vi "AdjustCorrectPosition.vi"(6 "Robot":refnum<class "Robot.lvclass">, 7 "Game":refnum<class "Game.lvclass">, 8 "error in (no error)":errorcluster, 9 "IsShoot?":bool, 10 "Position":dbl[](array[numeric]), 11 "Utilities in":refnum<class "Utilities.lvclass">) -> (0 "error out":errorcluster, 1 "AdjustPosition":dbl[](array[numeric]), 3 "Utilities out":refnum<class "Utilities.lvclass">)   [LabVIEW 2021, in "Utilities.lvclass"]
uses:
  Utilities.lvclass
  Game_class/Game.lvclass
  Robot_class/Robot.lvclass
  Team_class/OffensivePlay.ctl
  Game_class/Game.lvclass/Game.ctl
  Parameters_class/Parameters.lvclass/Parameters.ctl
  Team_class/Team.lvclass/Team.ctl
  Object_class/Object.lvclass/Object.ctl
  Object_class/Read x.vi
  Object_class/Read y.vi
  Game_class/Read FieldRef.vi
  Game_class/Read EnemyRef.vi
  Game_class/Read BallRef.vi
  Game_class/Read Parameters.lvclass.vi
  Game_class/Read NewParameters.vi
  Game_class/Read OffensiveTeam.vi
  Team_class/Read OffensivePlay.vi
  Parameters_class/Read DistanceArea.vi
  Parameters_class/Read DistanceStop.vi
  Ally_class/Ally.lvclass
  Field_class/Field.lvclass
  Enemy_class/Enemy.lvclass
  Ball_class/Ball.lvclass
  Parameters_class/Parameters.lvclass
panel:
  out "output variable":sgl
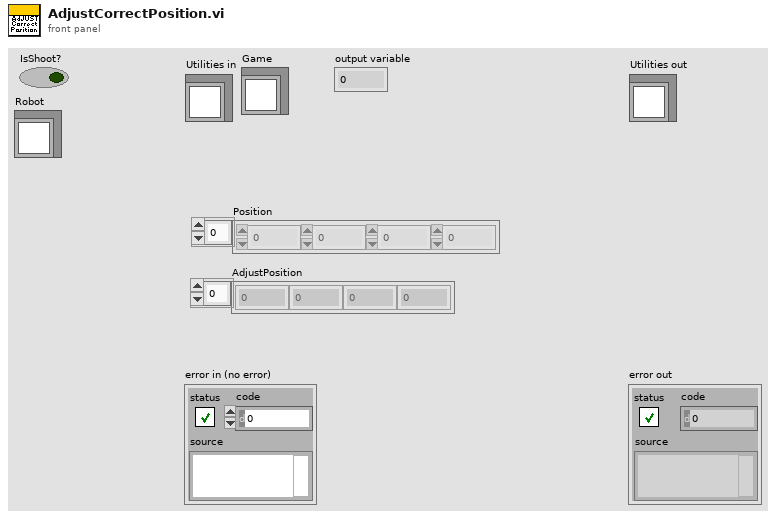
[diagram p1: front panel]
types:
  T1 = typedef "OffensivePlay.ctl" = enum16{"5RobotsPassGamePlay", "5PreparePassGame", "5RobotsKeeperGame", "KeeperPassToStriker", "5RobotsNormalGamePlay", "PrepareKeeperPass", "ACBPass", "ABCPass", "PrepareTriplePass", "TableWithStriker", "TableWith2ndStrikerPlay", "PrepareDoublePass", "PrepareRollToPass", "SimplePass", "PreparePass", "PassToStriker", "BallOutOfField", "PassTo2ndStriker", "StopOffensive", "Prepare Penalty Enemy", "EnemyPossessionAtEnemyField", "EnemyPossesionAtOurField", "TestPlay", "PreparePenaltyAlly", "KickPenaltyAlly", "PrepareKickoffAlly", "PrepareKickoffEnemy", "IndirectEnemy", "DirectEnemy", "PreparePassInGame1", "NormalGame", "DirectKick", "Pass", "Halt", "Timeout", "PassPlay", "PenaltyEnemy"}
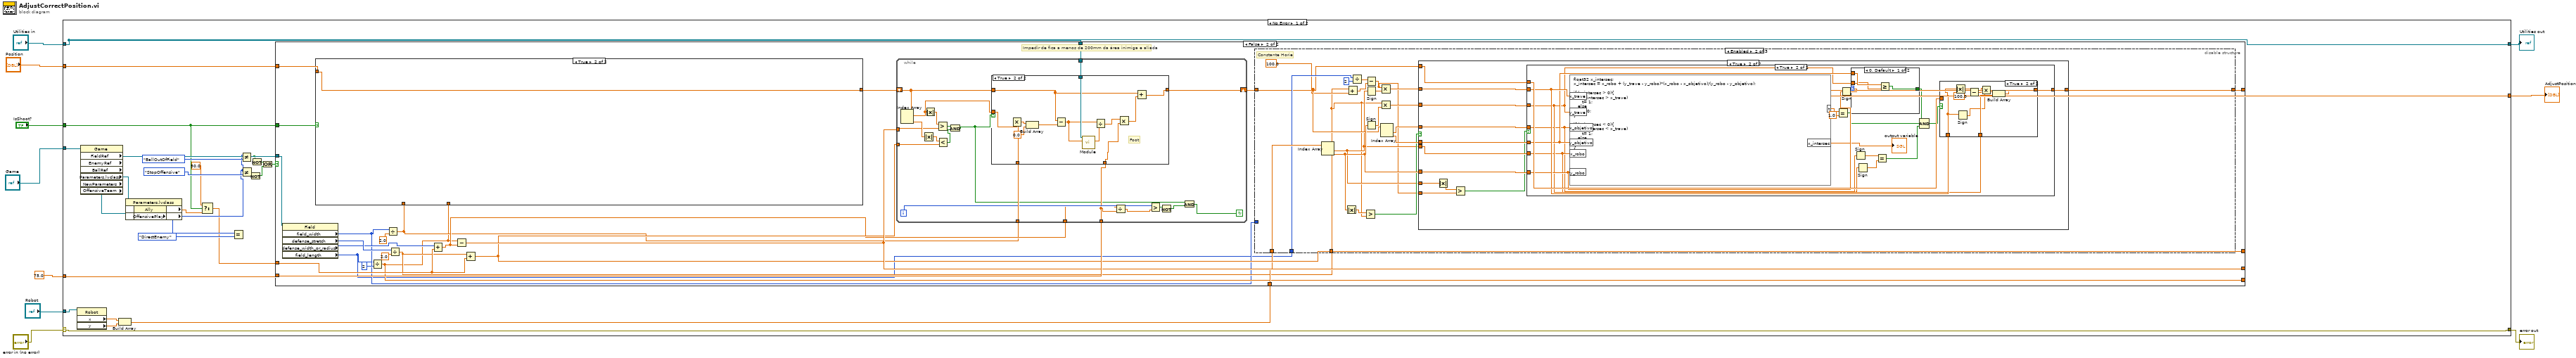
[diagram p0: block diagram]
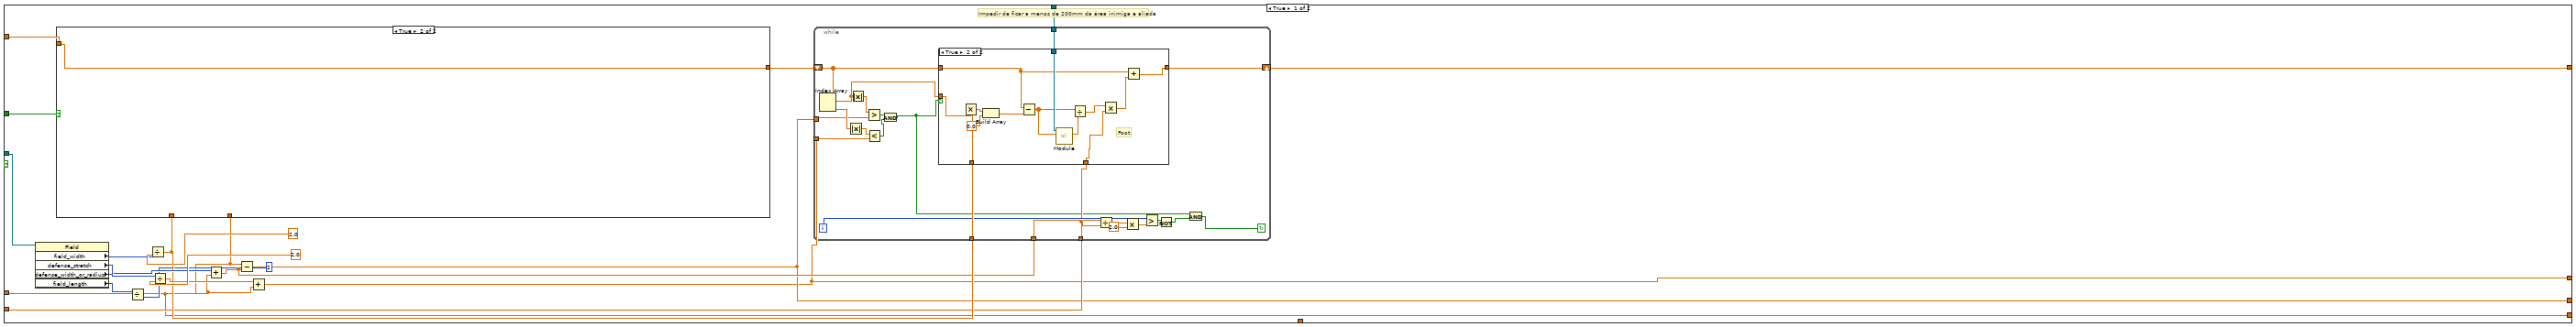
[diagram p2: hidden frame]
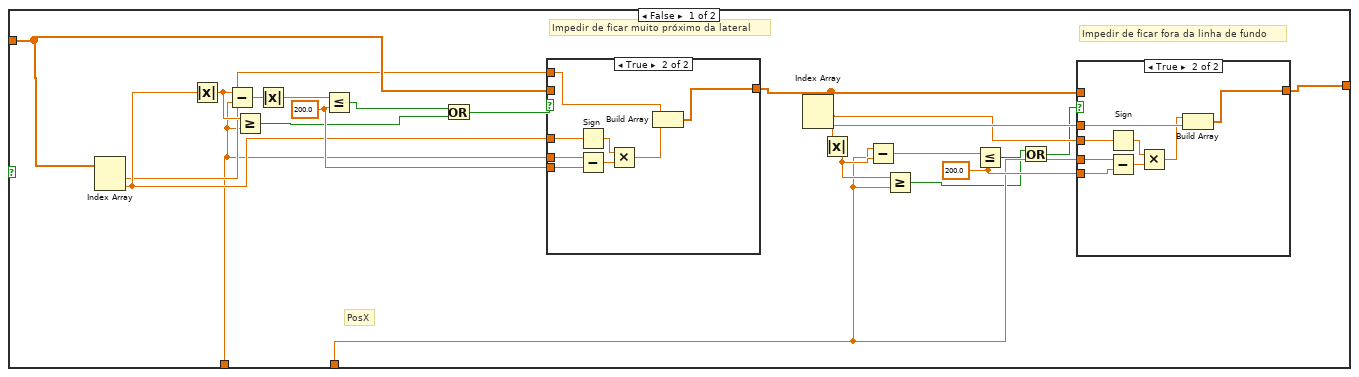
[diagram p3: hidden frame]
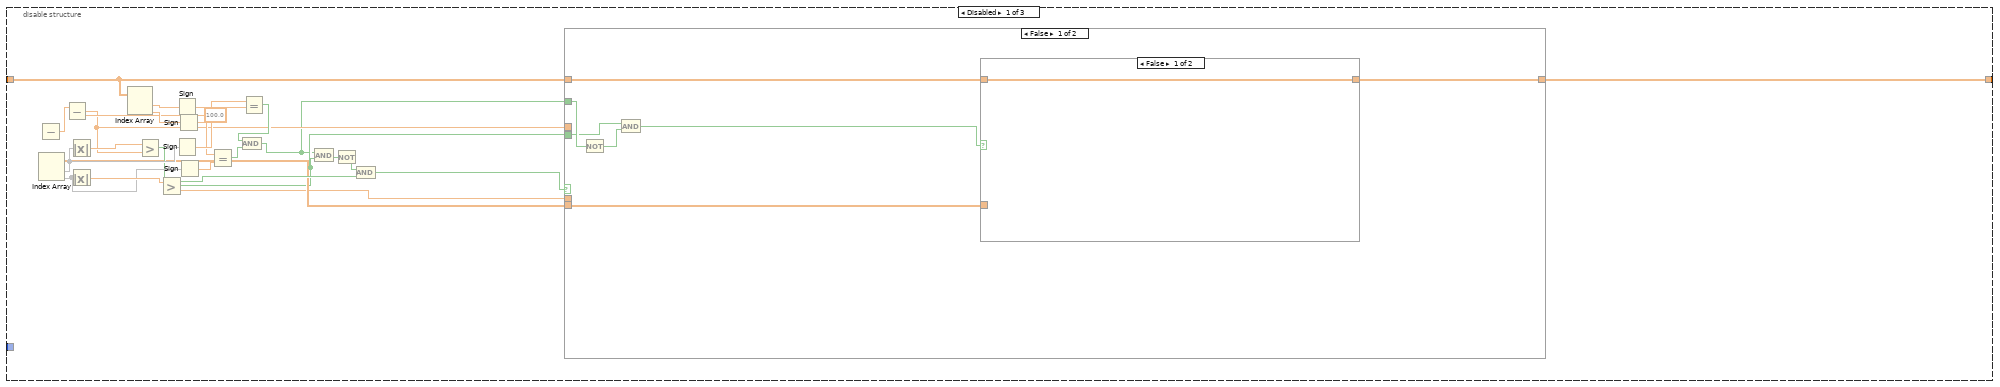
[diagram p7: hidden frame]
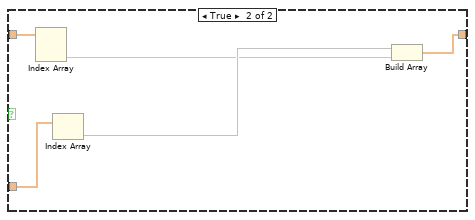
[diagram p8: hidden frame]
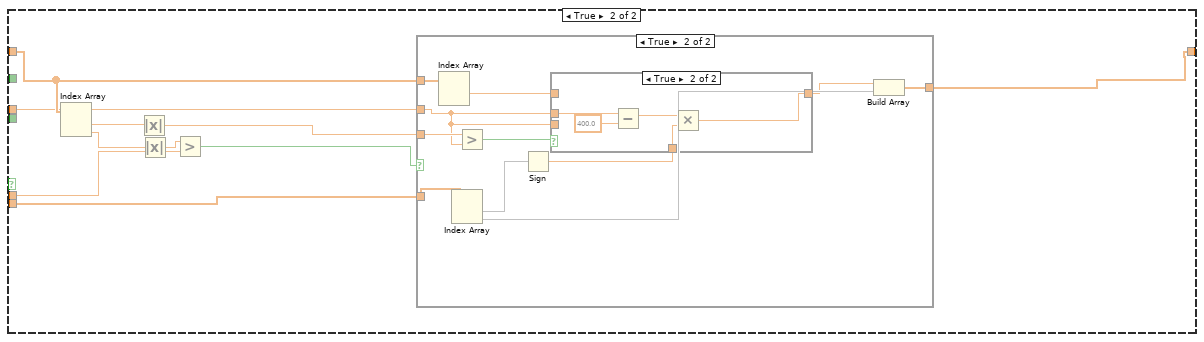
[diagram p9: hidden frame]
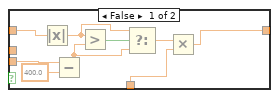
[diagram p11: hidden frame]
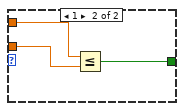
[diagram p14: hidden frame]
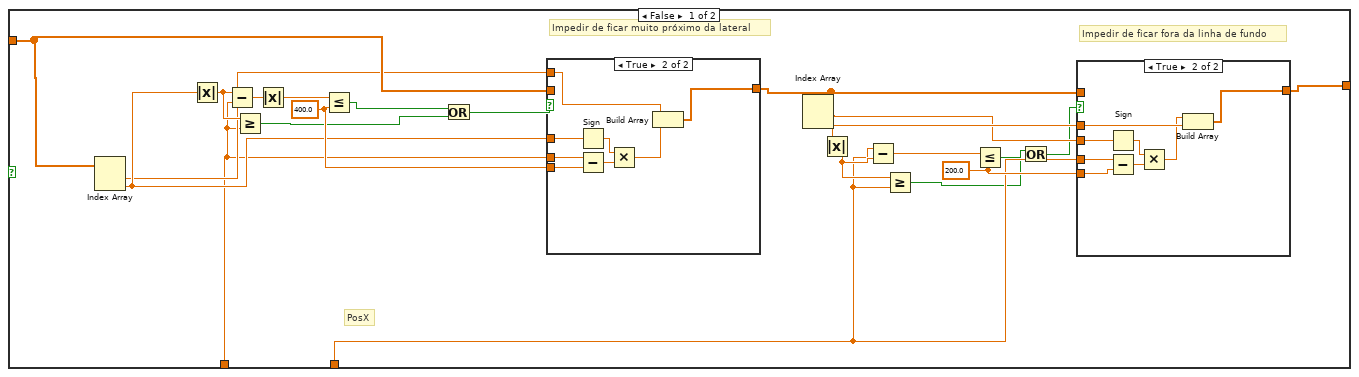
[diagram p17: hidden frame]
diagram:
  n1 = case shown="No Error" "error in (no error)" {
    selector: "error in (no error)" -> [w36 w377]
    tunnel: [w36 w377] -> w9
    tunnel: [w32 w376] -> w7
    tunnel: "Utilities in" -> [w32 w376]
    tunnel: "Position" -> [w35 _]
    tunnel: "Game" -> [w34 _]
    tunnel: [w15 _] -> w4
    tunnel: 75.0 ("element") -> [w31 _]
    tunnel: "IsShoot?" -> [w19 _]
    tunnel: "Robot" -> [w14 _]
    frame No Error {
      n2 = property class="Robot"(reference=w14) -> ("x"=w13:dbl, "y"=w12:dbl)  [unwired: 1 in, 2 out]
      n3 = property class="Game" props=["FieldRef", "EnemyRef", "BallRef", "Parameters.lvclass", "NewParameters", "OffensiveTeam"](reference=w34) -> ("FieldRef"=w33:refnum<class "Field.lvclass">, "Parameters.lvclass"=w30:refnum<class "Parameters.lvclass">, "OffensiveTeam"=w29:refnum<class "Ally.lvclass">)  [unwired: 1 in, 5 out]
      n4 = Build Array(w13, w12) -> (w11:dbl[])
      n5 = property class="Parameters.lvclass" props=["DistanceArea", "DistanceStop"](reference=w30) -> ("DistanceArea"=w18:dbl)  [unwired: 1 in, 3 out]
      n6 = property class="Ally"(reference=w29) -> ("OffensivePlay"=w21:T1)  [unwired: 1 in, 2 out]
      n7 = Select(t=50.0, s=w19, f=w18) -> (s? t:f=w16:dbl)
      n8 = Equal?(x=w21, y=OffensivePlay."DirectEnemy") -> ()  [unwired: 1 out]
      n9 = Not Equal?(x=w21, y=OffensivePlay."BallOutOfField") -> (x != y?=w25:bool)
      n10 = Not Equal?(x=w21, y=OffensivePlay."StopOffensive") -> (x != y?=w24:bool)
      n11 = Not(x=w24) -> (.not. x?=w22:bool)
      n12 = Not(x=w25) -> (.not. x?=w23:bool)
      n13 = Or(x=w23, y=w22) -> (x .or. y?=w26:bool)
      n14 = case shown="False" w26 {
        tunnel: w35 -> [w56 w156]
        tunnel: w33 -> [w55 w155]
        tunnel: [w48 w141] -> w15
        tunnel: w32 -> [w47 w153]
        tunnel: w31 -> [w46 w152]
        tunnel: w16 -> [w41 w148]
        tunnel: w19 -> [w40 w149]
        tunnel: [w39 w147] -> _
        tunnel: [w38 w145] -> _
        tunnel: [w37 w137] -> _
        tunnel: w11 -> [_ w140]
        frame True {
          # "Impedir de ficar a menos de 200mm da área inimiga e aliada"
          n15 = property class="Field"(reference=w55) -> ("field_width"=w54:i32, "defense_stretch"=w52:i32, "defense_width_or_radius"=w50:i32, "field_length"=w43:i32)  [unwired: 1 in, 2 out]
          n16 = Divide(x=w43, y=2) -> (x/y=w37:dbl)
          n17 = Divide(x=w54, y=2.0) -> (x/y=w49:dbl)
          n18 = case shown="True" w40 {
            tunnel: w56 -> [w72 w98]
            tunnel: w49 -> [w69 _]
            tunnel: [w68 w98] -> w44
            tunnel: w37 -> [w61 _]
            frame False {
              w65 = 200.0 ("y")
              w77 = 200.0 ("y")
              # "Impedir de ficar fora da linha de fundo"
              # "PosY"
              # "PosX"
              # "Impedir de ficar muito próximo da lateral"
              n19 = Index Array(array=w72) -> (element #1=w70:dbl, element #2=w71:dbl)  [unwired: 2 in]
              n20 = Absolute Value(x=w71) -> (abs(x)=w73:dbl)
              n21 = Subtract(x=w73, y=w69) -> (x-y=w79:dbl)
              n22 = Greater Or Equal?(x=w73, y=w69) -> (x >= y?=w74:bool)
              n23 = Absolute Value(x=w79) -> (abs(x)=w78:dbl)
              n24 = Less Or Equal?(x=w78, y=w77) -> (x <= y?=w75:bool)
              n25 = Or(x=w75, y=w74) -> (x .or. y?=w76:bool)
              n26 = case shown="True" w76 {
                tunnel: w70 -> [_ w97]
                tunnel: w69 -> [_ w96]
                tunnel: w77 -> [_ w95]
                tunnel: w71 -> [_ w92]
                tunnel: [w89 w90] -> w67
                tunnel: w72 -> [w89 _]
                frame False {
                }
                frame True {
                  n27 = Sign(1:w92) -> (0:w94:dbl)
                  n28 = Subtract(x=w96, y=w95) -> (x-y=w93:dbl)
                  n29 = Multiply(x=w94, y=w93) -> (x*y=w91:dbl)
                  n30 = Build Array(w97, w91) -> (w90:dbl[])
                }
              }
              n31 = Index Array(array=w67) -> (element #1=w64:dbl, element #2=w66:dbl)  [unwired: 2 in]
              n32 = Absolute Value(x=w64) -> (abs(x)=w62:dbl)
              n33 = Subtract(x=w61, y=w62) -> (x-y=w63:dbl)
              n34 = Greater Or Equal?(x=w62, y=w61) -> (x >= y?=w59:bool)
              n35 = Less Or Equal?(x=w63, y=w65) -> (x <= y?=w60:bool)
              n36 = Or(x=w60, y=w59) -> (x .or. y?=w58:bool)
              n37 = case shown="True" w58 {
                tunnel: [w80 w86] -> w68
                tunnel: w67 -> [w80 _]
                tunnel: w66 -> [_ w85]
                tunnel: w64 -> [_ w83]
                tunnel: w65 -> [_ w82]
                tunnel: w61 -> [_ w81]
                frame False {
                }
                frame True {
                  n38 = Sign(1:w83) -> (0:w88:dbl)
                  n39 = Subtract(x=w81, y=w82) -> (x-y=w87:dbl)
                  n40 = Multiply(x=w88, y=w87) -> (x*y=w84:dbl)
                  n41 = Build Array(w84, w85) -> (w86:dbl[])
                }
              }
            }
            frame True {
            }
          }
          n42 = Divide(x=w52, y=2.0) -> (x/y=w51:dbl)
          n43 = Add(x=w50, y=w41) -> (x+y=w45:dbl)
          n44 = Subtract(x=w37, y=w45) -> (x-y=w39:dbl)
          n45 = Add(x=w51, y=w41) -> (x+y=w38:dbl)
          n46 = while {
            tunnel: w49 -> [w120]
            tunnel: w47 -> [w119]
            tunnel: w39 -> [w106]
            tunnel: w38 -> [w118]
            shift-right: [w117] -> w48
            shift-left: w44 -> [w116]
            tunnel: w46 -> [w107]
            tunnel: w45 -> [w105]
            i -> [w109]
            stop <- w111 continue-if-true
            n47 = Index Array(array=w116) -> (element #1=w112:dbl, element #2=w113:dbl)  [unwired: 2 in]
            n48 = Absolute Value(x=w113) -> (abs(x)=w114:dbl)
            n49 = Absolute Value(x=w112) -> (abs(x)=w115:dbl)
            n50 = Greater?(x=w115, y=w106) -> (0:w104:bool)
            n51 = Less?(x=w114, y=w118) -> (x < y?=w103:bool)
            n52 = And(x=w104, y=w103) -> (x .and. y?=w102:bool)
            n53 = case shown="True" w102 {
              tunnel: [w121 w125] -> w117
              tunnel: w116 -> [w121 w126]
              tunnel: w120 -> [_ w133]
              tunnel: w119 -> [_ w131]
              tunnel: w112 -> [_ w124]
              tunnel: w107 -> [_ w122]
              frame False {
              }
              frame True {
                # "Foot"
                n54 = Multiply(x=w124, y=w133) -> (x*y=w132:dbl)
                n55 = Build Array(w132, 0.0 ("element")) -> (w123:dbl[])
                n56 = Subtract(x=w126, y=w123) -> (x-y=w130:dbl[])
                n57 = call "Module.vi"("2D vector"=w130, "Utilities in"=w131) -> ("Modulo"=w129:dbl)  [unwired: 7 in, 2 out]
                n58 = Divide(x=w130, y=w129) -> (x/y=w128:dbl[])
                n59 = Multiply(x=w128, y=w122) -> (x*y=w127:dbl[])
                n60 = Add(x=w126, y=w127) -> (x+y=w125:dbl[])
              }
            }
            n61 = Divide(x=w105, y=w107) -> (x/y=w101:dbl)
            n62 = Multiply(x=w101, y=2.0) -> (x*y=w99:dbl)
            n63 = Greater?(x=w109, y=w99) -> (0:w108:bool)
            n64 = Not(x=w108) -> (.not. x?=w110:bool)
            n65 = And(x=w102, y=w110) -> (x .and. y?=w111:bool)
          }
        }
        frame False {
          # "Impedir de fica a menos de 200mm da área inimiga e aliada"
          n66 = property class="Field"(reference=w155) -> ("field_width"=w136:i32, "defense_stretch"=w146:i32, "defense_width_or_radius"=w144:i32, "field_length"=w135:i32)  [unwired: 1 in, 2 out]
          n67 = Divide(x=w135, y=2) -> (x/y=w137:dbl)
          n68 = Divide(x=w136, y=2.0) -> (x/y=w138:dbl)
          n69 = case shown="True" w149 {
            tunnel: w156 -> [w315 w341]
            tunnel: w138 -> [w312 _]
            tunnel: [w311 w341] -> w151
            tunnel: w137 -> [w304 _]
            frame False {
              w308 = 200.0 ("y")
              w320 = 400.0 ("y")
              # "Impedir de ficar fora da linha de fundo"
              # "PosY"
              # "PosX"
              # "Impedir de ficar muito próximo da lateral"
              n70 = Index Array(array=w315) -> (element #1=w313:dbl, element #2=w314:dbl)  [unwired: 2 in]
              n71 = Absolute Value(x=w314) -> (abs(x)=w316:dbl)
              n72 = Subtract(x=w316, y=w312) -> (x-y=w322:dbl)
              n73 = Greater Or Equal?(x=w316, y=w312) -> (x >= y?=w317:bool)
              n74 = Absolute Value(x=w322) -> (abs(x)=w321:dbl)
              n75 = Less Or Equal?(x=w321, y=w320) -> (x <= y?=w318:bool)
              n76 = Or(x=w318, y=w317) -> (x .or. y?=w319:bool)
              n77 = case shown="True" w319 {
                tunnel: w313 -> [_ w340]
                tunnel: w312 -> [_ w339]
                tunnel: w320 -> [_ w338]
                tunnel: w314 -> [_ w335]
                tunnel: [w332 w333] -> w310
                tunnel: w315 -> [w332 _]
                frame False {
                }
                frame True {
                  n78 = Sign(1:w335) -> (0:w337:dbl)
                  n79 = Subtract(x=w339, y=w338) -> (x-y=w336:dbl)
                  n80 = Multiply(x=w337, y=w336) -> (x*y=w334:dbl)
                  n81 = Build Array(w340, w334) -> (w333:dbl[])
                }
              }
              n82 = Index Array(array=w310) -> (element #1=w307:dbl, element #2=w309:dbl)  [unwired: 2 in]
              n83 = Absolute Value(x=w307) -> (abs(x)=w305:dbl)
              n84 = Subtract(x=w304, y=w305) -> (x-y=w306:dbl)
              n85 = Greater Or Equal?(x=w305, y=w304) -> (x >= y?=w302:bool)
              n86 = Less Or Equal?(x=w306, y=w308) -> (x <= y?=w303:bool)
              n87 = Or(x=w303, y=w302) -> (x .or. y?=w301:bool)
              n88 = case shown="True" w301 {
                tunnel: [w323 w329] -> w311
                tunnel: w310 -> [w323 _]
                tunnel: w309 -> [_ w328]
                tunnel: w307 -> [_ w326]
                tunnel: w308 -> [_ w325]
                tunnel: w304 -> [_ w324]
                frame False {
                }
                frame True {
                  n89 = Sign(1:w326) -> (0:w331:dbl)
                  n90 = Subtract(x=w324, y=w325) -> (x-y=w330:dbl)
                  n91 = Multiply(x=w331, y=w330) -> (x*y=w327:dbl)
                  n92 = Build Array(w327, w328) -> (w329:dbl[])
                }
              }
            }
            frame True {
            }
          }
          n93 = Divide(x=w146, y=2.0) -> (x/y=w139:dbl)
          n94 = Add(x=w144, y=w148) -> (x+y=w143:dbl)
          n95 = Subtract(x=w137, y=w143) -> (x-y=w147:dbl)
          n96 = Add(x=w139, y=w148) -> (x+y=w145:dbl)
          n97 = while {
            tunnel: w138 -> [w361]
            tunnel: w153 -> [w360]
            tunnel: w147 -> [w347]
            tunnel: w145 -> [w359]
            shift-right: [w358] -> w142
            shift-left: w151 -> [w357]
            tunnel: w152 -> [w348]
            tunnel: w143 -> [w346]
            i -> [w350]
            stop <- w352 continue-if-true
            n98 = Index Array(array=w357) -> (element #1=w353:dbl, element #2=w354:dbl)  [unwired: 2 in]
            n99 = Absolute Value(x=w354) -> (abs(x)=w355:dbl)
            n100 = Absolute Value(x=w353) -> (abs(x)=w356:dbl)
            n101 = Greater?(x=w356, y=w347) -> (0:w345:bool)
            n102 = Less?(x=w355, y=w359) -> (x < y?=w344:bool)
            n103 = And(x=w345, y=w344) -> (x .and. y?=w343:bool)
            n104 = case shown="True" w343 {
              tunnel: [w362 w366] -> w358
              tunnel: w357 -> [w362 w367]
              tunnel: w361 -> [_ w374]
              tunnel: w360 -> [_ w372]
              tunnel: w353 -> [_ w365]
              tunnel: w348 -> [_ w363]
              frame False {
              }
              frame True {
                # "Foot"
                n105 = Multiply(x=w365, y=w374) -> (x*y=w373:dbl)
                n106 = Build Array(w373, 0.0 ("element")) -> (w364:dbl[])
                n107 = Subtract(x=w367, y=w364) -> (x-y=w371:dbl[])
                n108 = call "Module.vi"("2D vector"=w371, "Utilities in"=w372) -> ("Modulo"=w370:dbl)  [unwired: 7 in, 2 out]
                n109 = Divide(x=w371, y=w370) -> (x/y=w369:dbl[])
                n110 = Multiply(x=w369, y=w363) -> (x*y=w368:dbl[])
                n111 = Add(x=w367, y=w368) -> (x+y=w366:dbl[])
              }
            }
            n112 = Divide(x=w346, y=w348) -> (x/y=w342:dbl)
            n113 = Greater?(x=w350, y=w342) -> (0:w349:bool)
            n114 = Not(x=w349) -> (.not. x?=w351:bool)
            n115 = And(x=w343, y=w351) -> (x .and. y?=w352:bool)
          }
          n116 = disable-structure shown="Enabled" {
            disable-tunnel: w142 -> [w164 w240 _]
            disable-tunnel: [w166 w239 _] -> w141
            disable-tunnel: w140 -> [_ w253 _]
            disable-tunnel: w139 -> [_ w234 _]
            disable-tunnel: w136 -> [_ _ _]
            disable-tunnel: w135 -> [_ w252 _]
            frame Disabled {
              n117 = Subtract() -> (x=w163:dbl, y=w162:dbl, x-y=w169:dbl)
              n118 = Subtract(x=w169, y=100.0) -> (x-y=w167:dbl)
              n119 = Index Array(array=w164) -> (element #1=w182:dbl, element #2=w181:dbl)  [unwired: 2 in]
              n120 = Sign(1:w182) -> (0:w175:dbl)
              n121 = Sign(1:w181) -> (0:w174:dbl)
              n122 = Index Array(array=w165) -> (element #1=w180, element #2=w179)  [unwired: 2 in]
              n123 = Absolute Value(x=w180) -> (abs(x)=w183:dbl)
              n124 = Absolute Value(x=w179) -> (abs(x)=w184:dbl)
              n125 = Greater?(x=w183, y=w167) -> (0:w172:bool)
              n126 = Greater?(x=w184) -> (y=w161:dbl, 0:w159:bool)
              n127 = Sign(1:w180) -> (0:w176:dbl)
              n128 = Sign(1:w179) -> (0:w173:dbl)
              n129 = Equal?(x=w174, y=w173) -> (x = y?=w178:bool)
              n130 = Equal?(x=w176, y=w175) -> (x = y?=w177:bool)
              n131 = And(x=w177, y=w178) -> (x .and. y?=w158:bool)
              n132 = And(x=w158, y=w159) -> (x .and. y?=w171:bool)
              n133 = Not(x=w171) -> (.not. x?=w170:bool)
              n134 = And(x=w170, y=w172) -> (x .and. y?=w160:bool)
              n135 = case shown="False" w160 {
                tunnel: w164 -> [w190 w205]
                tunnel: [w189 w207] -> w166
                tunnel: [w188 w206] -> w165
                tunnel: w167 -> [_ w204]
                tunnel: w161 -> [_ w202]
                tunnel: w159 -> [w185 _]
                tunnel: w158 -> [w186 _]
                frame False {
                  n136 = Not(x=w186) -> (.not. x?=w191:bool)
                  n137 = And(x=w185, y=w191) -> (x .and. y?=w187:bool)
                  n138 = case shown="False" w187 {
                    tunnel: w190 -> [w192 w194]
                    tunnel: [w192 w197] -> w189
                    tunnel: w188 -> [_ w196]
                    frame False {
                    }
                    frame True {
                      n139 = Index Array(array=w194) -> (element #2=w193:dbl)  [unwired: 2 in, 1 out]
                      n140 = Index Array(array=w196) -> (element=w195)  [unwired: 1 in]
                      n141 = Build Array(w195, w193) -> (w197:dbl[])
                    }
                  }
                }
                frame True {
                  n142 = Index Array(array=w205) -> (element #1=w200:dbl, element #2=w203:dbl)  [unwired: 2 in]
                  n143 = Absolute Value(x=w200) -> (abs(x)=w199:dbl)
                  n144 = Absolute Value(x=w203) -> (abs(x)=w201:dbl)
                  n145 = Greater?(x=w201, y=w202) -> (0:w198:bool)
                  n146 = case shown="True" w198 {
                    tunnel: w205 -> [w208 w219]
                    tunnel: [w208 w218] -> w207
                    tunnel: w206 -> [_ w217]
                    tunnel: w204 -> [_ w209]
                    tunnel: w199 -> [_ w211]
                    frame False {
                    }
                    frame True {
                      n147 = Index Array(array=w219) -> (element #1=w215:dbl)  [unwired: 2 in, 1 out]
                      n148 = Index Array(array=w217) -> (element #1=w213, element #2=w216)  [unwired: 2 in]
                      n149 = Greater?(x=w211, y=w209) -> (0:w210:bool)
                      n150 = Sign(1:w213) -> (0:w212:dbl)
                      n151 = case shown="True" w210 {
                        tunnel: w215 -> [w228 _]
                        tunnel: [w220 w229] -> w214
                        tunnel: w209 -> [_ w233]
                        tunnel: w212 -> [w222 w231]
                        tunnel: w209 -> [w227 _]
                        frame False {
                          n152 = Absolute Value(x=w228) -> (abs(x)=w225:dbl)
                          n153 = Subtract(x=w227, y=400.0) -> (x-y=w224:dbl)
                          n154 = Greater?(x=w225, y=w224) -> (0:w223:bool)
                          n155 = Select(t=w225, s=w223, f=w224) -> (s? t:f=w221:dbl)
                          n156 = Multiply(x=w221, y=w222) -> (x*y=w220:dbl)
                        }
                        frame True {
                          n157 = Subtract(x=w233, y=400.0) -> (x-y=w230:dbl)
                          n158 = Multiply(x=w230, y=w231) -> (x*y=w229:dbl)
                        }
                      }
                      n159 = Build Array(w214, w216) -> (w218:dbl[])
                    }
                  }
                }
              }
            }
            frame Enabled {
              # "Constante Horie"
              n160 = Index Array(array=w253) -> (element #1=w238:dbl, element #2=w243:dbl)  [unwired: 2 in]
              n161 = Absolute Value(x=w243) -> (abs(x)=w242:dbl)
              n162 = Add(x=w234, y=100.0) -> (x+y=w235:dbl)
              n163 = Divide(x=w252, y=2) -> (x/y=w248:dbl)
              n164 = Greater?(x=w242, y=w234) -> (0:w241:bool)
              n165 = Subtract(x=w248, y=w235) -> (x-y=w237:dbl)
              n166 = Sign(1:w238) -> (0:w250:dbl)
              n167 = Sign(1:w243) -> (0:w249:dbl)
              n168 = Multiply(x=w237, y=w250) -> (x*y=w247:dbl)
              n169 = Multiply(x=w234, y=w249) -> (x*y=w246:dbl)
              n170 = Index Array(array=w240) -> (element #1=w245:dbl, element #2=w244:dbl)  [unwired: 2 in]
              n171 = case shown="True" w241 {
                tunnel: w247 -> [_ w266]
                tunnel: w246 -> [_ w265]
                tunnel: w245 -> [_ w264]
                tunnel: w244 -> [_ w263]
                tunnel: w238 -> [_ w262]
                tunnel: w243 -> [_ w261]
                tunnel: w240 -> [w254 w256]
                tunnel: [w254 w255] -> w239
                tunnel: w238 -> [_ w259]
                tunnel: w237 -> [_ w258]
                frame False {
                }
                frame True {
                  n172 = Absolute Value(x=w259) -> (abs(x)=w260:dbl)
                  n173 = Greater?(x=w260, y=w258) -> (0:w257:bool)
                  n174 = case shown="True" w257 {
                    tunnel: w266 -> [_ w281]
                    tunnel: w265 -> [_ w277]
                    tunnel: w264 -> [_ w274]
                    tunnel: w263 -> [_ w278]
                    tunnel: w262 -> [_ w275]
                    tunnel: w261 -> [_ w279]
                    tunnel: w256 -> [w267 w282]
                    tunnel: [w267 w283] -> w255
                    frame False {
                    }
                    frame True {
                      n175 = formula code="float32 x_intersec;\nx_intersec = x_robo + (y_trave - y_robo)*(x_robo - x_objetivo)/(y_robo - y_objetivo);\n\nif (x_intersec > 0){\n   if(x_intersec > x_trave)\n      t= 1;\n   else\n      t=0;\n}\n\nif (x_intersec < 0){\n   if(x_intersec < x_trave)\n      t= 1;\n   else\n      t=0;\n}"("x_trave"=w281, "y_trave"=w277, "x_objetivo"=w274, "y_objetivo"=w278, "x_robo"=w275, "y_robo"=w279) -> ("t"=w285:dbl, "x_intersec"=→"output variable":sgl)
                      n176 = Equal?(x=w285, y=1.0) -> (x = y?=w269:bool)
                      n177 = Sign(1:w279) -> (0:w280:dbl)
                      n178 = case shown="0, Default" w280 {
                        tunnel: w278 -> [w288 w291]
                        tunnel: w277 -> [w287 w290]
                        tunnel: [w286 w289] -> w271
                        frame 0, Default {
                          n179 = Greater Or Equal?(x=w288, y=w287) -> (x >= y?=w286:bool)
                        }
                        frame 1 {
                          n180 = Less Or Equal?(x=w291, y=w290) -> (x <= y?=w289:bool)
                        }
                      }
                      n181 = Sign(1:w275) -> (0:w273:dbl)
                      n182 = Sign(1:w274) -> (0:w272:dbl)
                      n183 = Equal?(x=w273, y=w272) -> (x = y?=w270:bool)
                      n184 = Compound Arithmetic op=AND(w271, w269, w270) -> (w268:bool)
                      n185 = case shown="True" w268 {
                        tunnel: [w292 w299] -> w283
                        tunnel: w282 -> [w292 _]
                        tunnel: w281 -> [_ w295]
                        tunnel: w277 -> [_ w300]
                        frame False {
                        }
                        frame True {
                          n186 = Absolute Value(x=w295) -> (abs(x)=w298:dbl)
                          n187 = Sign(1:w295) -> (0:w294:dbl)
                          n188 = Subtract(x=w298, y=100.0) -> (x-y=w296:dbl)
                          n189 = Multiply(x=w296, y=w294) -> (x*y=w293:dbl)
                          n190 = Build Array(w293, w300) -> (w299:dbl[])
                        }
                      }
                    }
                  }
                }
              }
            }
            frame Disabled {
            }
          }
        }
      }
    }
    frame Error {
    }
  }
  "error out" <- w9
  "Utilities out" <- w7
  "AdjustPosition" <- w4
